vi "Get Properties.vi"(8 "error in (no error)":errorcluster, 11 "Device Reference In":T2 format="%.0x") -> (0 "error out":errorcluster, 1 "Enable OVP":bool, 2 "ID Query?":bool, 3 "Device Reference Out":T2 format="%.0x", 4 "Voltage Limit":dbl, 5 "Update Rate":u16, 6 "VISA Resource Name":string, 7 "serial":T1={"Baud Rate"=9600, "Parity"=0, "Data Bits"=8, "Stop Bits"=10} {"Baud Rate" items=["1200"=1200, "2400"=2400, "4800"=4800, "9600"=9600]; "Parity" items=["None", "Odd", "Even"]; "Data Bits" items=["7"=7, "8"=8]; "Stop Bits" items=["1.0"=10]})   [LabVIEW 2011, in "BK Precision 91xx (GPIB) Custom Device.lvlib"]
uses:
  BK Precision 91xx (GPIB) Custom Device.lvlib
  <vilib>/NI Veristand/Custom Device API/Custom Device Item Ref.ctl
  Serial Config.ctl
  Global Strings.vi
  <vilib>/NI Veristand/Custom Device API/Get Item Property (String).vi
  <vilib>/NI Veristand/Custom Device API/Get Item Property (Boolean).vi
  <vilib>/NI Veristand/Custom Device API/Get Item Property (Double).vi
  <vilib>/NI Veristand/Custom Device API/Get Item Property (U16).vi
  <vilib>/NI Veristand/Custom Device API/Get Item Property (Variant).vi
  <vilib>/NI Veristand/Custom Device API/Custom Device API.lvlib
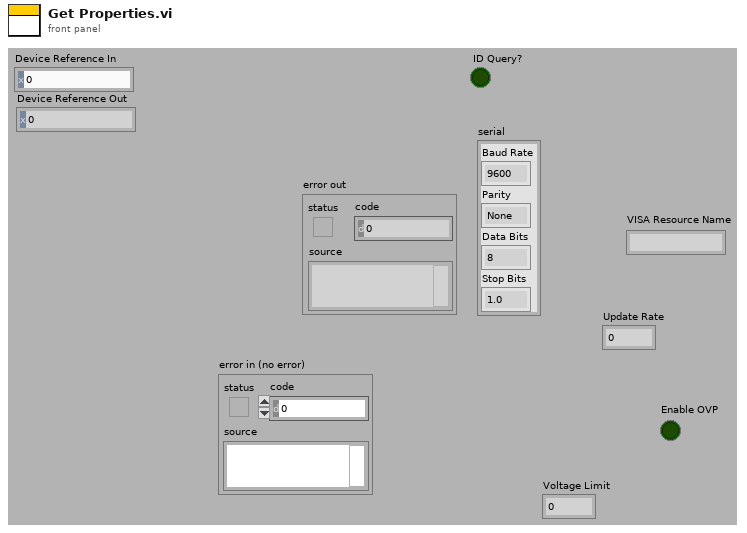
[diagram p1: front panel]
types:
  T1 = typedef "BK Precision 91xx (GPIB) Custom Device.lvlib/Serial Config.ctl" = cluster{"Baud Rate":u32, "Parity":u16, "Data Bits":u16, "Stop Bits":u16}
  T2 = typedef "Custom Device API.lvlib/Custom Device Item Ref.ctl" = u64
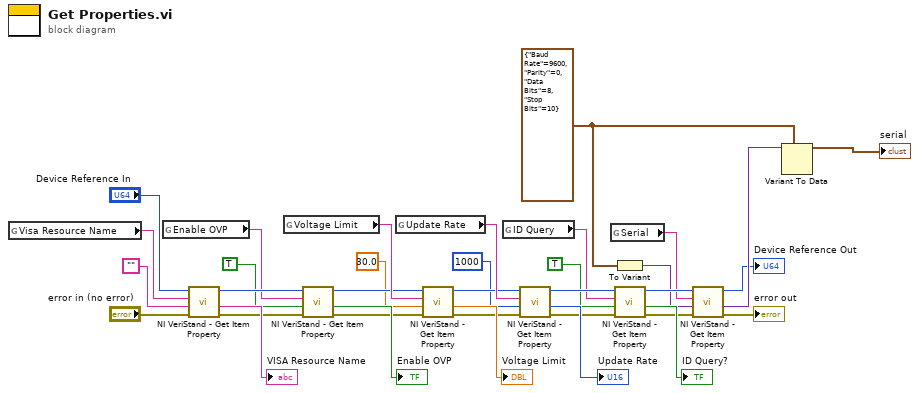
[diagram p0: block diagram]
diagram:
  w3 = T1 {"Baud Rate"=9600, "Parity"=0, "Data Bits"=8, "Stop Bits"=10} ("Serial Configuration")
  n1 = global read "Global Strings.vi" "Visa Resource Name"() -> (w32:string)
  n2 = global read "Global Strings.vi" "Enable OVP"() -> (w28:string)
  n3 = call-poly <vilib>:"NI VeriStand - Get Item Property.vi"("error in (no error)"="error in (no error)", "Default Value"="", "Property Name"=w32, "Item Ref in"="Device Reference In") -> ("error out"=w30:errorcluster, "Value"=→"VISA Resource Name":string, "Item Ref out"=w29:T2)  [unwired: 4 in, 1 out]
  n4 = global read "Global Strings.vi" "Voltage Limit"() -> (w26:string)
  n5 = call-poly <vilib>:"NI VeriStand - Get Item Property.vi"("error in (no error)"=w30, "Default Value"=TRUE, "Property Name"=w28, "Item Ref in"=w29) -> ("error out"=w25:errorcluster, "Value"=→"Enable OVP":bool, "Item Ref out"=w24:T2)  [unwired: 4 in, 1 out]
  n6 = global read "Global Strings.vi" "Update Rate"() -> (w21:string)
  n7 = call-poly <vilib>:"NI VeriStand - Get Item Property.vi"("error in (no error)"=w25, "Default Value"=30.0, "Property Name"=w26, "Item Ref in"=w24) -> ("error out"=w22:errorcluster, "Value"=→"Voltage Limit":dbl, "Item Ref out"=w20:T2)  [unwired: 4 in, 1 out]
  n8 = global read "Global Strings.vi" "ID Query"() -> (w16:string)
  n9 = call-poly <vilib>:"NI VeriStand - Get Item Property.vi"("error in (no error)"=w22, "Default Value"=u16 1000, "Property Name"=w21, "Item Ref in"=w20) -> ("error out"=w18:errorcluster, "Value"=→"Update Rate":u16, "Item Ref out"=w17:T2)  [unwired: 4 in, 1 out]
  n10 = global read "Global Strings.vi" "Serial"() -> (w7:string)
  n11 = To Variant(anything=w3) -> (Variant=w6:variant)
  n12 = call-poly <vilib>:"NI VeriStand - Get Item Property.vi"("error in (no error)"=w18, "Default Value"=TRUE, "Property Name"=w16, "Item Ref in"=w17) -> ("error out"=w9:errorcluster, "Value"=→"ID Query?":bool, "Item Ref out"=w8:T2)  [unwired: 4 in, 1 out]
  n13 = call-poly <vilib>:"NI VeriStand - Get Item Property.vi"("error in (no error)"=w9, "Default Value"=w6, "Property Name"=w7, "Item Ref in"=w8) -> ("error out"=→"error out":errorcluster, "Value"=w5:variant, "Item Ref out"=→"Device Reference Out":T2)  [unwired: 4 in, 1 out]
  n14 = Variant To Data(type=w3, Variant=w5) -> (data=→"serial":T1)  [unwired: 1 in, 1 out]
